vi "Check Status (No Objects) - Spectrometer.vi"(8 "error in (no error)":errorcluster, 11 "Cluster In":T4) -> (0 "error out":errorcluster, 1 "Status":string, 2 "Ready?":bool, 3 "Cluster Out":T4)   [LabVIEW 2012]
doc: "Checks if the instrument is powered on and updates its member data with the instrument's current status."
uses:
  JY-SPEX-TRIAX/controls.llb/Monochromator System Number.ctl
  JY-SPEX-TRIAX/controls.llb/Mirror Position.ctl
  JY-SPEX-TRIAX/controls.llb/Turret Position (TRIAX).ctl
  JY-SPEX-TRIAX/controls.llb/Slits.ctl
  Global/GPIB Numbers.vi
  JY-SPEX-TRIAX/JY-SPEX-TRIAX.lvlib
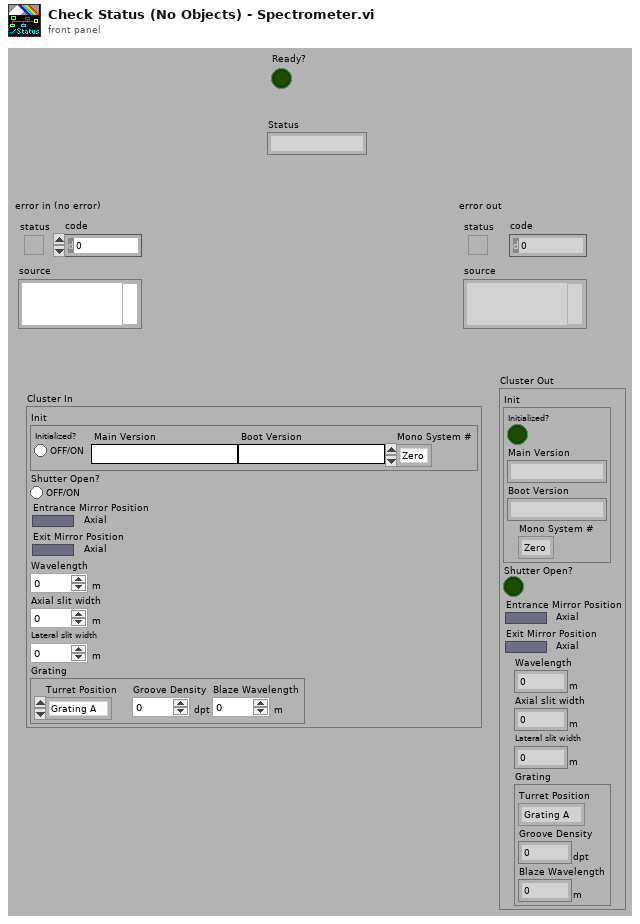
[diagram p1: front panel]
types:
  T1 = typedef "JY-SPEX-TRIAX.lvlib/Monochromator System Number.ctl" = enum16{"Zero", "One"}
  T2 = typedef "JY-SPEX-TRIAX.lvlib/Mirror Position.ctl" = bool
  T3 = typedef "JY-SPEX-TRIAX.lvlib/Turret Position (TRIAX).ctl" = enum16{"Grating A", "Grating B", "Grating C"}
  T4 = cluster{"Init":cluster{"Initialized?":bool, "Main Version":string, "Boot Version":string, "Mono System #":T1}, "Shutter Open?":bool, "Entrance Mirror Position":T2, "Exit Mirror Position":T2, "Wavelength":dbl[unit], "Axial slit width":dbl[unit], "Lateral slit width":dbl[unit], "Grating":cluster{"Turret Position":T3, "Groove Density":dbl[unit], "Blaze Wavelength":dbl[unit]}}
  T5 = typedef "GPIB Type Def.ctl" = cluster{"Name":string, "bus":dbl, "GPIB":dbl, "GPIB as string":string, "byte":i32, "VISA Resource Name":refnum<visa-resource-name>}
  T6 = typedef "JY-SPEX-TRIAX.lvlib/Slits.ctl" = enum16{"0 (Front/Axial Entrance)", "1 (Side/Lateral Entrance)", "2 (Front/Axial Exit)", "3 (Side/Lateral Exit)"}
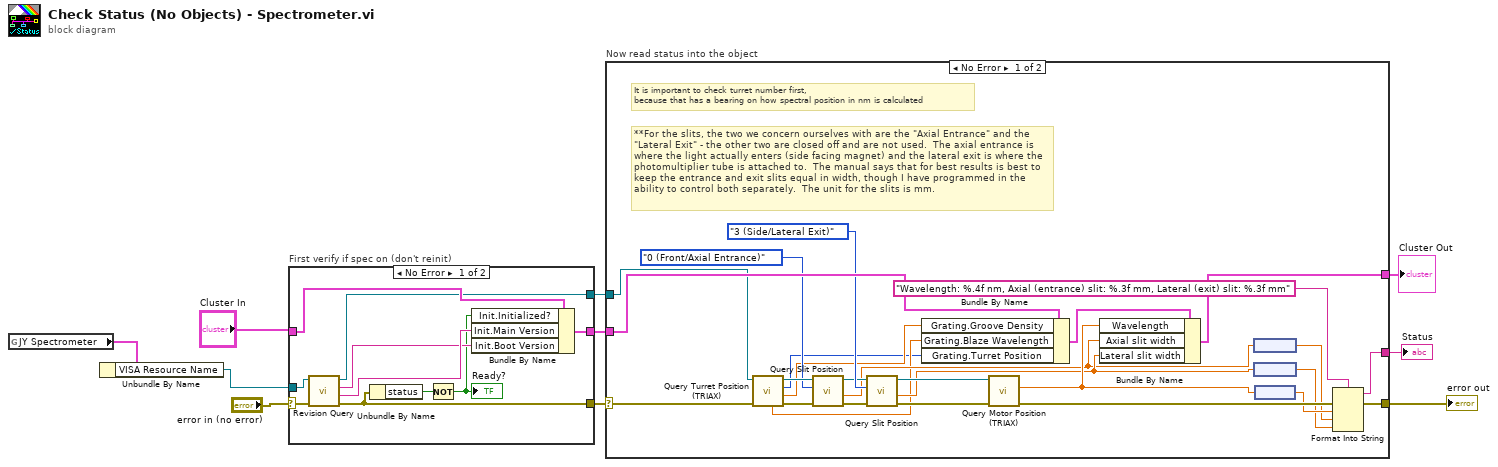
[diagram p0: block diagram]
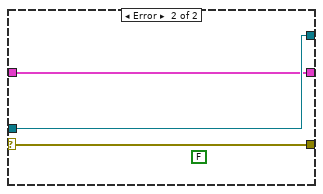
[diagram p2: hidden frame]
diagram:
  n1 = global read "GPIB Numbers.vi" "JY Spectrometer"() -> (w6:T5)
  n2 = Unbundle By Name(w6) -> ("VISA Resource Name"=w4:refnum<visa-resource-name>)
  n3 = case "First verify if spec on (don't reinit)" shown="No Error" "error in (no error)" {
    selector: "error in (no error)" -> [w16 w23]
    tunnel: [w20 w21] -> w9
    tunnel: "Cluster In" -> [w19 w21]
    tunnel: w4 -> [w18 w22]
    tunnel: [w17 w23] -> w8
    tunnel: [w14 w22] -> w7
    frame No Error {
      n4 = call "Revision Query.vi"("error in (no error)"=w16, "VISA resource name"=w18) -> ("error out"=w17:errorcluster, "Main Firmware Revision"=w13:string, "Boot Firmware Revision"=w12:string, "VISA resource name out"=w14:refnum<visa-resource-name>)  [unwired: 6 out]
      n5 = Unbundle By Name(w17) -> ("status"=w15:bool)
      n6 = Not(x=w15) -> (.not. x?=w11:bool)
      "Ready?" <- w11
      n7 = Bundle By Name(cluster=w19, "Init.Initialized?"=w11, "Init.Main Version"=w13, "Init.Boot Version"=w12) -> (w20:T4)
    }
    frame Error {
      (unwired) FALSE ("status")
    }
  }
  n8 = case "Now read status into the object" shown="No Error" w8 {
    selector: w8 -> [w30 w50]
    tunnel: w9 -> [w45 w51]
    tunnel: [w44 w51] -> w1
    tunnel: [w47 w50] -> w2
    tunnel: [w46 _] -> w10
    tunnel: w7 -> [w43 _]
    frame No Error {
      # "**For the slits, the two we concern ourselves with are the \"Axial Entrance\" and the \"Lateral Exit\" - the other two are closed off and are not used.  The axial entrance is where the light actually enters (side facing magnet) and the lateral exit is where the photomultiplier tube is attached to.  The manual says that for best results is best to keep the entrance and exit slits equal in width, though I have programmed in the ability to control both separately.  The unit for the slits is mm."
      # "It is important to check turret number first, \nbecause that has a bearing on how spectral position in nm is calculated"
      n9 = call "Query Turret Position (TRIAX).vi"("error in (no error)"=w30, "VISA resource name"=w43) -> ("error out"=w41:errorcluster, "Groove Density"=w29:dbl[unit], "Turret Position"=w27:T3, "VISA resource name out"=w42:refnum<visa-resource-name>, "Blaze Wavelength"=w28:dbl[unit])  [unwired: 1 in, 4 out]
      n10 = call "Query Slit Position.vi"("error in (no error)"=w41, "Slit (Front/Axial Entrance)"=Slits."0 (Front/Axial Entrance)", "VISA resource name"=w42) -> ("error out"=w38:errorcluster, "Slit Position"=w31:dbl[unit], "VISA resource name out"=w37:refnum<visa-resource-name>)  [unwired: 1 in, 5 out]
      n11 = call "Query Slit Position.vi"("error in (no error)"=w38, "Slit (Front/Axial Entrance)"=Slits."3 (Side/Lateral Exit)", "VISA resource name"=w37) -> ("error out"=w35:errorcluster, "Slit Position"=w32:dbl[unit], "VISA resource name out"=w36:refnum<visa-resource-name>)  [unwired: 1 in, 5 out]
      n12 = Bundle By Name(cluster=w45, "Grating.Groove Density"=w29, "Grating.Blaze Wavelength"=w28, "Grating.Turret Position"=w27) -> (w48:T4)
      n13 = call "Query Motor Position (TRIAX).vi"("error in (no error)"=w35, "VISA resource name"=w36) -> ("error out"=w34:errorcluster, "wavelength"=w33:dbl[unit])  [unwired: 1 in, 7 out]
      n14 = Bundle By Name(cluster=w48, "Wavelength"=w33, "Axial slit width"=w31, "Lateral slit width"=w32) -> (w44:T4)
      n15 = node(w31) -> (w25:dbl)
      n16 = node(w32) -> (w24:dbl)
      n17 = node(w33) -> (w26:dbl)
      n18 = Format Into String(format string="Wavelength: %.4f nm, Axial (entrance) slit: %.3f mm, Lateral (exit) slit: %.3f mm", error in=w34, w26, w25, w24) -> (resulting string=w46:string, error out=w47:errorcluster)  [unwired: 1 in]
    }
    frame Error {
    }
  }
  "error out" <- w2
  "Status" <- w10
  "Cluster Out" <- w1
